vi "breadth_first_search_(BFS).vi"(8 "error in (no error)":errorcluster, 10 "starting-nodes ([]: top-level nodes)":refnum<class "Node.lvclass">[](array[class]), 11 "DiGraph in":refnum<class "DiGraph.lvclass">) -> (0 "error out":errorcluster, 2 "nodes (by visit order)":refnum<class "Node.lvclass">[](array[class]))   [LabVIEW 2020, in "graph.lvlib" / "DiGraph.lvclass"]
uses:
  DiGraph.lvclass
  C:/Projects/labview-project-load-tools/source/submodules/graph-api-labview/source/api/Graph/Graph.lvclass
  Node/Node.lvclass
  ID/ID.lvclass
  DiGraph.lvclass/DiGraph.ctl
  Graph/Graph.lvclass/Graph.ctl
  Node/Node.lvclass/Node.ctl
  ac1f2d44-9eb7-4ef7-81be-08fc9f061da4.vi
  Graph/Graph.lvclass
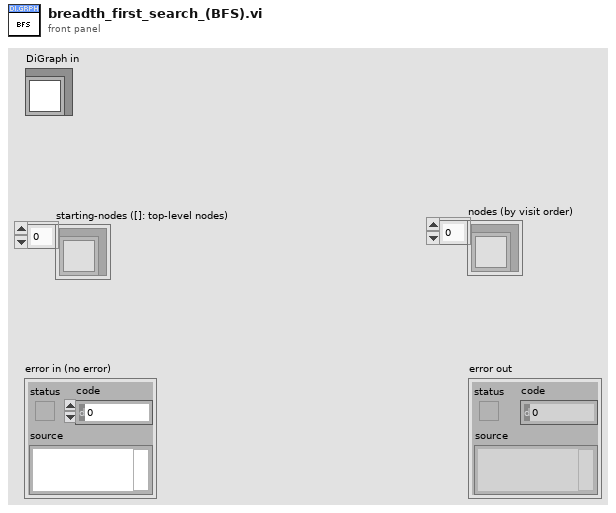
[diagram p1: front panel]
types:
  T1 = map{refnum<class "ID.lvclass">, set{refnum<class "ID.lvclass">}}
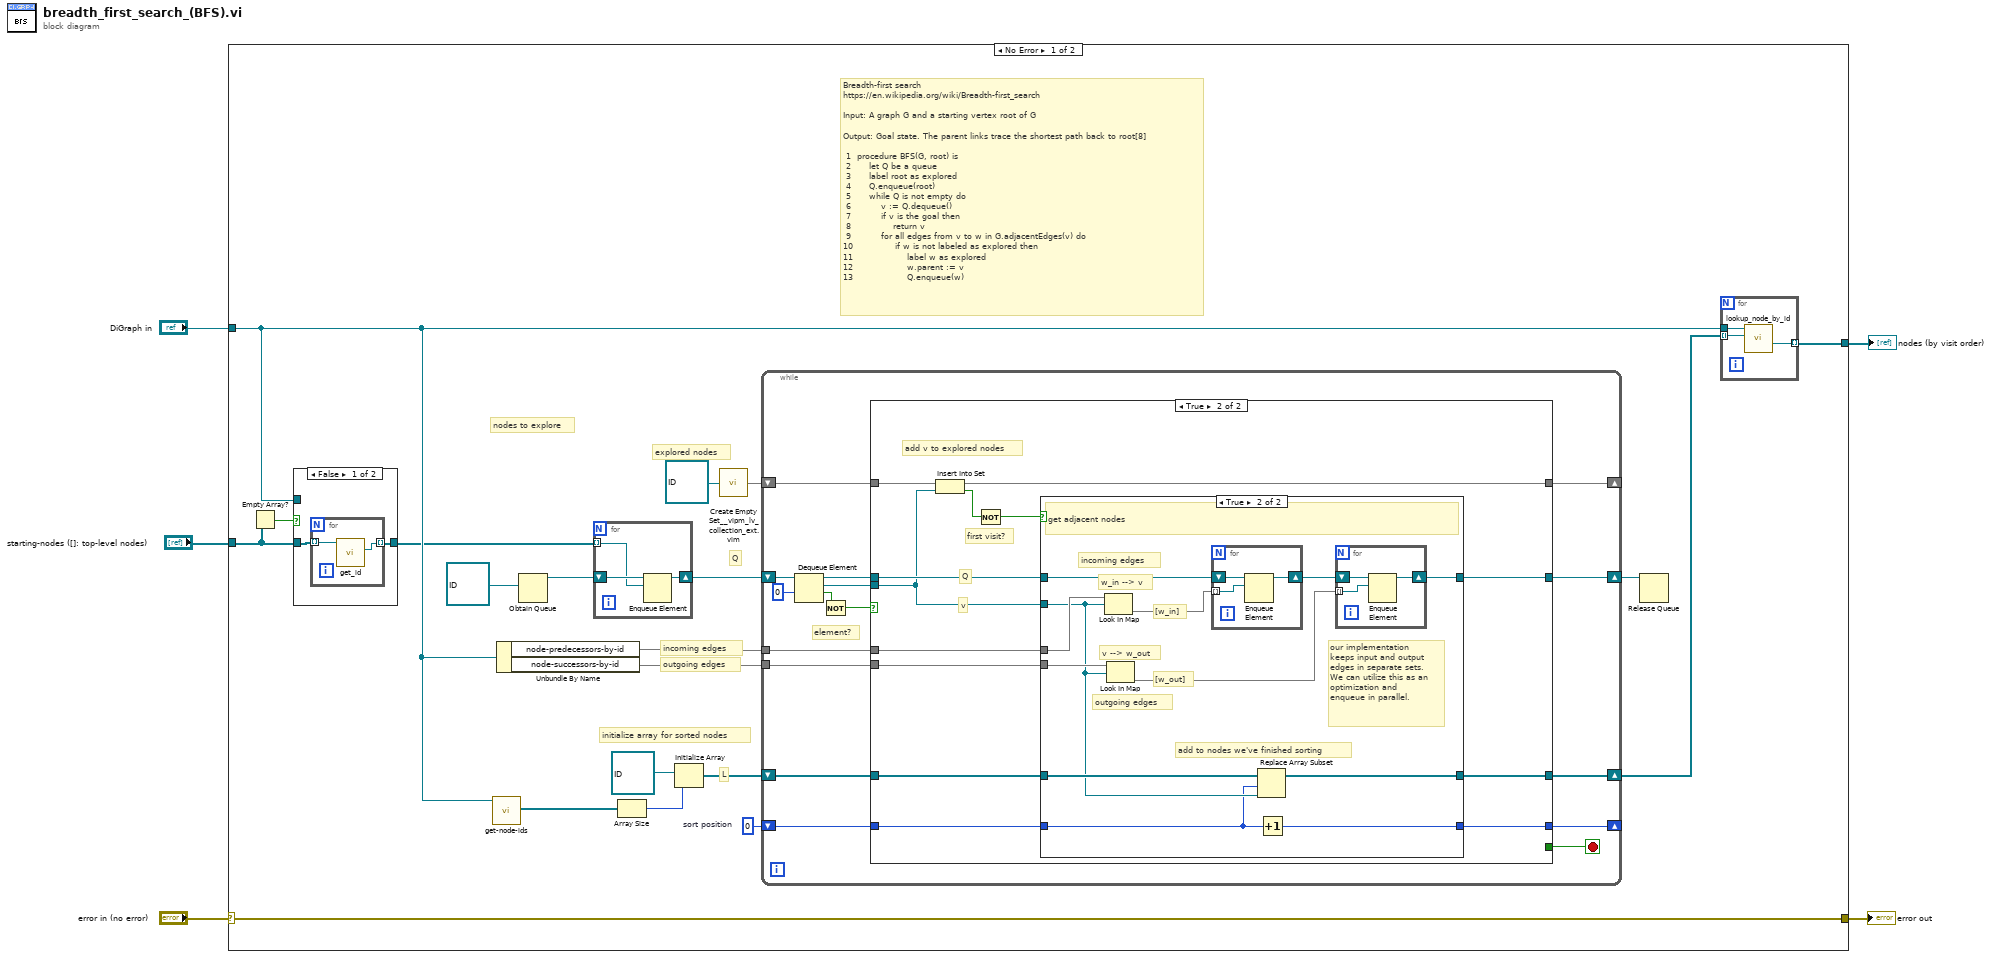
[diagram p0: block diagram]
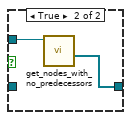
[diagram p2: hidden frame]
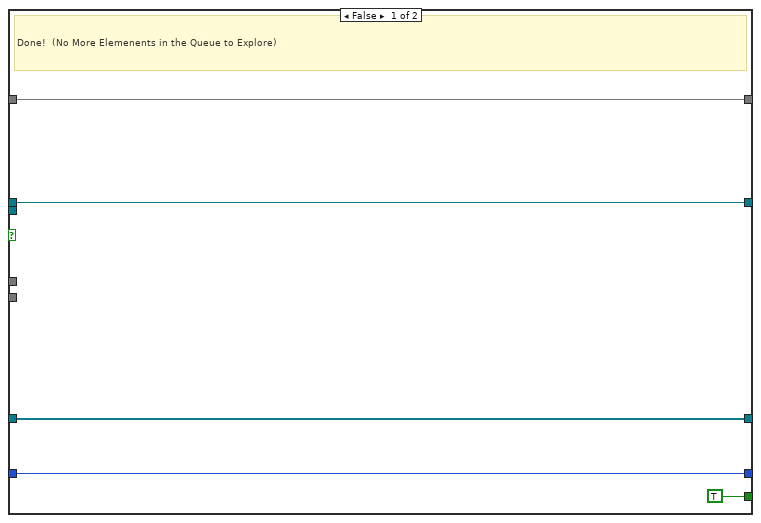
[diagram p3: hidden frame]
diagram:
  n1 = case shown="No Error" "error in (no error)" {
    selector: "error in (no error)" -> [w10 w93]
    tunnel: [w10 w93] -> w4
    tunnel: "DiGraph in" -> [w8 _]
    tunnel: [w15 _] -> w2
    tunnel: "starting-nodes ([]: top-level nodes)" -> [w6 _]
    frame No Error {
      w25 = 0  # sort position
      # "Q"
      # "explored nodes"
      # "initialize array for sorted nodes"
      # "Breadth-first search\nhttps://en.wikipedia.org/wiki/Breadth-first_search\n\nInput: A graph G and a starting vertex root of G\n\nOutput: Goal state. The parent links trace the shortest path back to root[8]\n\n 1  procedure BFS(G, root) is\n 2      let Q be a queue\n 3      label root as explored\n 4      Q.enqueue(root)\n 5      while Q is not empty do\n 6          v := Q.dequeue()\n 7          if v is the goal then\n 8              return v\n 9          for all edges from v to w in G.adjacentEdges(v) do\n10              if w is not labeled as explored then\n11                  label w as explored\n12                  w.parent := v\n13                  Q.enqueue(w)"
      # "outgoing edges"
      # "incoming edges"
      # "L"
      # "nodes to explore"
      n2 = Empty Array?(array=w6) -> (empty?=w9:bool)
      n3 = case shown="False" w9 {
        tunnel: w8 -> [_ w31]
        tunnel: [w27 w30] -> w7
        tunnel: w6 -> [w26 _]
        frame False {
          n4 = for {
            tunnel: w26 -> [w29] mode=indexing
            tunnel: [w28] -> w27 mode=indexing
            n5 = call "get_id.vi"("node"=w29) -> ("node-id"=w28:refnum<class "ID.lvclass">)  [unwired: 9 in, 1 out]
          }
        }
        frame True {
          n6 = call "get_nodes_with_no_predecessors.vi"("DiGraph in"=w31) -> ("node-ids (no predecessors)"=w30:refnum<class "ID.lvclass">[])  [unwired: 10 in]
        }
      }
      n7 = call "get-node-ids.vi"("Graph in"=w8) -> ("node-ids"=w22:refnum<class "ID.lvclass">[])  [unwired: 10 in]
      n8 = Unbundle By Name(w8) -> ("node-predecessors-by-id"=w18:T1, "node-successors-by-id"=w17:T1)
      n9 = Obtain Queue(element data type=refnum<class "ID.lvclass"> refnum ("node-id")) -> (queue out=w14:refnum<queue>)  [unwired: 4 in, 2 out]
      n10 = for {
        shift-right: [w33] -> w13
        shift-left: w14 -> [w34]
        tunnel: w7 -> [w32] mode=indexing
        n11 = Enqueue Element(queue=w34, element=w32) -> (queue out=w33:refnum<queue>)  [unwired: 2 in, 2 out]
      }
      n12 = Array Size(array=w22) -> (size(s)=w23:i32)
      n13 = Initialize Array(refnum<class "ID.lvclass"> refnum ("node-id"), w23) -> (w24:refnum<class "ID.lvclass">[])
      n14 = call "Create Empty Set__vipm_lv_collection_ext.vim"("element type"=refnum<class "ID.lvclass"> refnum ("node")) -> ("empty set"=w21:set{refnum<class "ID.lvclass">})  [unwired: 6 in]
      n15 = while {
        shift-right: [w47] -> w16
        shift-left: w24 -> [w50]
        shift-right: [w39] -> w12
        shift-left: w13 -> [w42]
        shift-right: [w48] -> _
        shift-left: w25 -> [w49]
        shift-right: [w45] -> _
        shift-left: w21 -> [w46]
        tunnel: w18 -> [w44]
        tunnel: w17 -> [w43]
        stop <- w35 stop-if-true
        # "element?"
        n16 = Dequeue Element(queue=w42, timeout in ms (-1)=0) -> (queue out=w40:refnum<queue>, element=w41:refnum<class "ID.lvclass">, timed out?=w37:bool)  [unwired: 1 in, 1 out]
        n17 = Not(x=w37) -> (.not. x?=w36:bool)
        n18 = case shown="True" w36 {
          tunnel: w50 -> [w53 w60]
          tunnel: w49 -> [w54 w58]
          tunnel: [w54 w56] -> w48
          tunnel: [w53 w57] -> w47
          tunnel: w46 -> [w51 w68]
          tunnel: [w51 w67] -> w45
          tunnel: w44 -> [_ w65]
          tunnel: w43 -> [_ w64]
          tunnel: w41 -> [_ w59]
          tunnel: w40 -> [w52 w63]
          tunnel: [w52 w62] -> w39
          tunnel: [TRUE _] -> w35
          frame False {
            # "Done!  (No More Elemenents in the Queue to Explore)"
          }
          frame True {
            # "v"
            # "Q"
            # "first visit?"
            # "add v to explored nodes"
            n19 = Insert Into Set(10:w59, 11:w68) -> (2:w66:bool, 3:w67:set{refnum<class "ID.lvclass">})
            n20 = Not(x=w66) -> (.not. x?=w61:bool)
            n21 = case shown="True" w61 {
              tunnel: w63 -> [w71 w74]
              tunnel: [w71 w72] -> w62
              tunnel: w59 -> [_ w77]
              tunnel: w65 -> [_ w83]
              tunnel: w64 -> [_ w82]
              tunnel: w60 -> [w70 w79]
              tunnel: w58 -> [w69 w76]
              tunnel: [w70 w78] -> w57
              tunnel: [w69 w75] -> w56
              frame False {
                # "do nothing - already visited"
              }
              frame True {
                # "our implementation keeps input and output edges in separate sets. We can utilize this as an optimization and enqueue in parallel."
                # "v --> w_out"
                # "w_in --> v"
                # "add to nodes we've finished sorting"
                # "incoming edges"
                # "[w_in]"
                # "[w_out]"
                # "outgoing edges"
                # "get adjacent nodes"
                n22 = Look In Map(map=w83, key=w77) -> (value=w81:set{refnum<class "ID.lvclass">})  [unwired: 1 in, 1 out]
                n23 = Look In Map(map=w82, key=w77) -> (value=w80:set{refnum<class "ID.lvclass">})  [unwired: 1 in, 1 out]
                n24 = for {
                  shift-right: [w88] -> w73
                  shift-left: w74 -> [w89]
                  tunnel: w81 -> [w87] mode=indexing
                  n25 = Enqueue Element(queue=w89, element=w87) -> (queue out=w88:refnum<queue>)  [unwired: 2 in, 2 out]
                }
                n26 = Replace Array Subset(array=w79, new element=w77, index=w76) -> (w78:refnum<class "ID.lvclass">[])
                n27 = Increment(x=w76) -> (x+1=w75:i32)
                n28 = for {
                  shift-right: [w85] -> w72
                  shift-left: w73 -> [w86]
                  tunnel: w80 -> [w84] mode=indexing
                  n29 = Enqueue Element(queue=w86, element=w84) -> (queue out=w85:refnum<queue>)  [unwired: 2 in, 2 out]
                }
              }
            }
          }
        }
      }
      n30 = Release Queue(queue=w12) -> ()  [unwired: 2 in, 3 out]
      n31 = for {
        tunnel: w8 -> [w92]
        tunnel: w16 -> [w91] mode=indexing
        tunnel: [w90] -> w15 mode=indexing
        n32 = call "lookup_node_by_id.vi"("node_id"=w91, "graph"=w92) -> ("node"=w90:refnum<class "Node.lvclass">)  [unwired: 8 in, 1 out]
      }
    }
    frame Error {
    }
  }
  "error out" <- w4
  "nodes (by visit order)" <- w2
